vi "GetLimsTestSteps.vi"(8 "error in (no error)":errorcluster, 10 "test-id":i32, 11 "ByteQXAPIBase in":refnum<class "ByteQXAPIBase.lvclass">) -> (0 "error out":errorcluster, 2 "list of steps":T1[](array[typedef]), 3 "ByteQXAPIBase out":refnum<class "ByteQXAPIBase.lvclass">)   [LabVIEW 2019, in "ByteQXWebAPI.lvlib" / "ByteQXAPIBase.lvclass"]
doc: "Obtain the list of steps for a Test based on the test-id"
uses:
  ByteQXAPIBase.lvclass
  TypeDef/Step.ctl
  TypeDef/Asset.ctl
  Private/module.ctl
  ByteQXAPIBase.lvclass/ByteQXAPIBase.ctl
  <vilib>/Bytelabs/ByteREST/ByteRESTClass/ByteRESTBase/RESTBase.lvclass
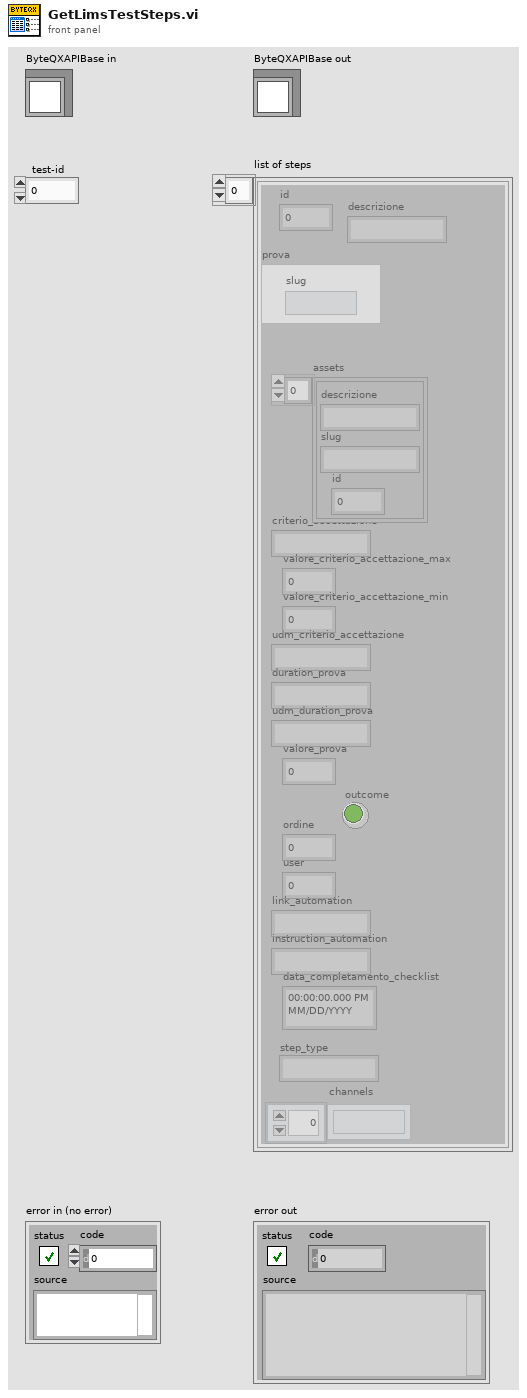
[diagram p1: front panel]
types:
  T1 = typedef "ByteQXWebAPI.lvlib/ByteQXAPIBase.lvclass/Step.ctl" = cluster{"id":i32, "descrizione":string, "prova":cluster{"slug":string}, "assets":T2[], "criterio_accettazione":string, "valore_criterio_accettazione_max":dbl, "valore_criterio_accettazione_min":dbl, "udm_criterio_accettazione":string, "duration_prova":string, "udm_duration_prova":string, "valore_prova":dbl, "ordine":i32, "user":i32, "link_automation":string, "instruction_automation":string, "data_completamento_checklist":timestamp, "outcome":bool, "step_type":string, "channels":string[]}
  T2 = typedef "ByteQXWebAPI.lvlib/ByteQXAPIBase.lvclass/Asset.ctl" = cluster{"descrizione":string, "slug":string, "id":i32}
  T3 = typedef "ByteQXWebAPI.lvlib/ByteQXAPIBase.lvclass/module.ctl" = enum16{"gs", "tms"}
  T4 = cluster{"id":i32, "descrizione":string, "prova":cluster{"slug":string}, "assets":T2[], "criterio_accettazione":string, "valore_criterio_accettazione_max":dbl, "valore_criterio_accettazione_min":dbl, "udm_criterio_accettazione":string, "duration_prova":string, "udm_duration_prova":string, "data_completamento_checklist":string, "valore_prova":dbl, "outcome":string, "ordine":i32, "user":i32, "link_automation":string, "instruction_automation":string}[]
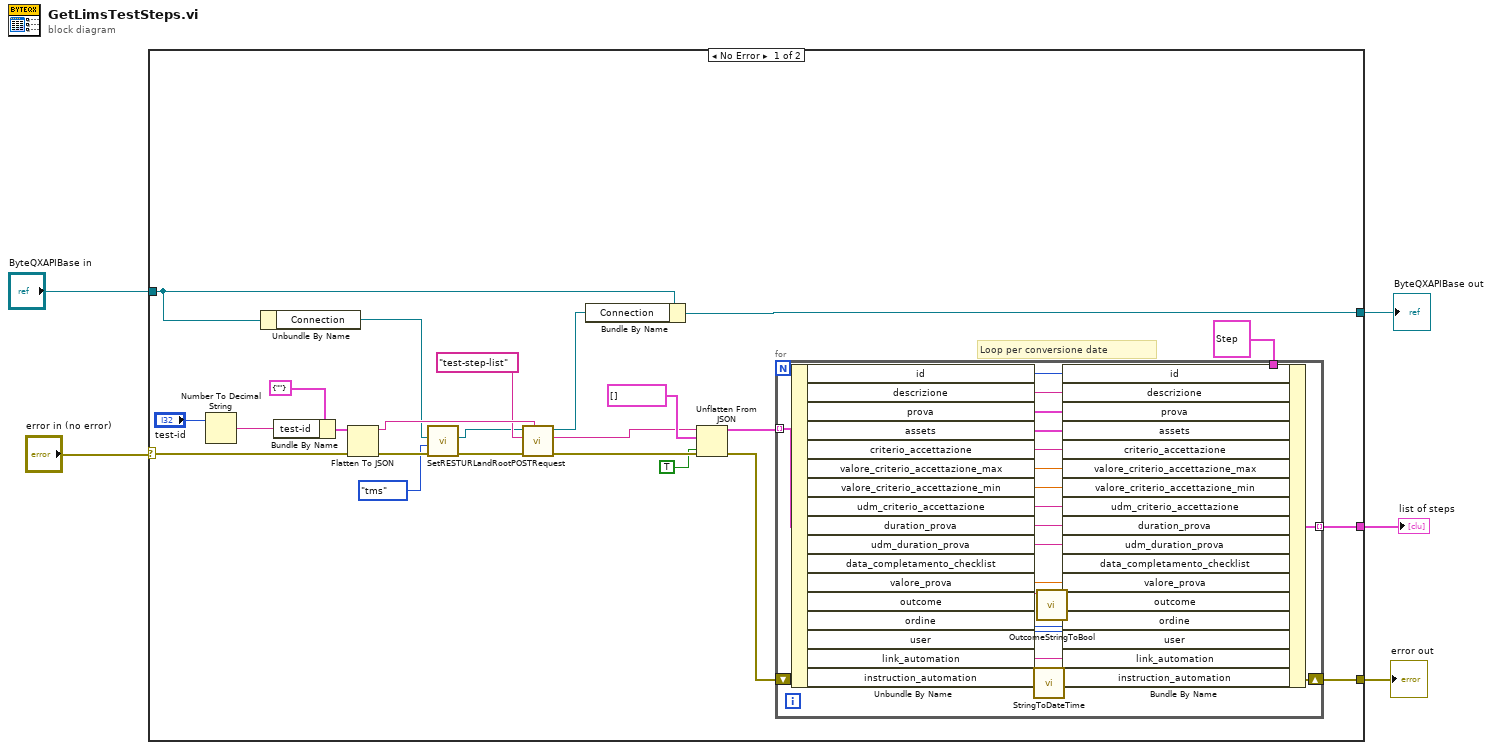
[diagram p0: block diagram]
diagram:
  n1 = case shown="No Error" "error in (no error)" {
    selector: "error in (no error)" -> [w28 w55]
    tunnel: [w13 w55] -> w4
    tunnel: [w29 w54] -> w2
    tunnel: "ByteQXAPIBase in" -> [w20 w54]
    tunnel: [w11 _] -> w1
    frame No Error {
      # "Loop per conversione date"
      n2 = Number To Decimal String(number="test-id") -> (decimal integer string=w18:string)  [unwired: 1 in]
      n3 = Unbundle By Name(w20) -> ("Connection"=w8:refnum<class "RESTBase.lvclass">)
      n4 = Bundle By Name(cluster=cluster{"test-id":string} {"test-id"=""} ("Request"), "test-id"=w18) -> (w17:cluster{"test-id":string})
      n5 = Flatten To JSON(anything=w17, error in (no error)=w28) -> (JSON string=w26:string, 11:w10:errorcluster)  [unwired: 1 in]
      n6 = call "SetRESTURLandRoot.vi"("error in (no error)"=w10, "module"=module."tms", "ByteREST in"=w8) -> ("error out"=w9:errorcluster, "ByteREST out"=w7:refnum<class "RESTBase.lvclass">)  [unwired: 7 in]
      n7 = call-dynamic "POSTRequest.vi"("Body in"=w26, "error in (no error)"=w9, "Request"="test-step-list", "ByteRESTBase in"=w7) -> ("error out"=w24:errorcluster, "Body"=w22:string, "ByteRESTBase out"=w23:refnum<class "RESTBase.lvclass">)  [unwired: 4 in, 1 out]
      n8 = Bundle By Name(cluster=w20, "Connection"=w23) -> (w29:refnum<class "ByteQXAPIBase.lvclass">)
      n9 = Unflatten From JSON(JSON string=w22, type and defaults=T4 [], default null elements? (F)=TRUE, error in (no error)=w24) -> (value=w16:T4, error out=w14:errorcluster)  [unwired: 3 in]
      n10 = for {
        tunnel: w16 -> [w53] mode=indexing
        tunnel: T1 {"id"=0, "descrizione"="", "prova"={"slug"=""}, "assets"=[], "criterio_accettazione"="", "valore_criterio_accettazione_max"=0.0, "valore_criterio_accettazione_min"=0.0, "udm_criterio_accettazione"="", "duration_prova"="", "udm_duration_prova"="", "valore_prova"=0.0, "ordine"=0, "user"=0, "link_automation"="", "instruction_automation"="", "data_completamento_checklist"=timestamp(0 s since 1904-01-01), "outcome"=FALSE, "step_type"="", "channels"=[]} -> [w52]
        shift-right: [w33] -> w13
        shift-left: w14 -> [w34]
        tunnel: [w32] -> w11 mode=indexing
        n11 = Unbundle By Name(w53) -> ("id"=w51:i32, "descrizione"=w50:string, "prova"=w49:cluster{"slug":string}, "assets"=w48:T2[], "criterio_accettazione"=w47:string, "valore_criterio_accettazione_max"=w46:dbl, "valore_criterio_accettazione_min"=w45:dbl, "udm_criterio_accettazione"=w44:string, "duration_prova"=w43:string, "udm_duration_prova"=w42:string, "data_completamento_checklist"=w41:string, "valore_prova"=w39:dbl, "outcome"=w31:string, "ordine"=w38:i32, "user"=w37:i32, "link_automation"=w36:string, "instruction_automation"=w35:string)
        n12 = call "StringToDateTime.vi"("error in (no error)"=w34, "datetime string"=w41) -> ("error out"=w33:errorcluster, "timestamp"=w40:timestamp)  [unwired: 8 in]
        n13 = call "OutcomeStringToBool.vi"("outcome string"=w31) -> ("outcome bool"=w30:bool)  [unwired: 10 in]
        n14 = Bundle By Name(cluster=w52, "id"=w51, "descrizione"=w50, "prova"=w49, "assets"=w48, "criterio_accettazione"=w47, "valore_criterio_accettazione_max"=w46, "valore_criterio_accettazione_min"=w45, "udm_criterio_accettazione"=w44, "duration_prova"=w43, "udm_duration_prova"=w42, "data_completamento_checklist"=w40, "valore_prova"=w39, "outcome"=w30, "ordine"=w38, "user"=w37, "link_automation"=w36, "instruction_automation"=w35) -> (w32:T1)
      }
    }
    frame Error {
    }
  }
  "error out" <- w4
  "ByteQXAPIBase out" <- w2
  "list of steps" <- w1
